vi "test_libssh2_userauth_authenticated.vi"() -> ()   [LabVIEW 2017, in "integration_tests.lvlib"]
uses:
  integration_tests.lvlib
  libssh2/libssh2_session_handshake_tcp.vi
  libssh2/libssh2_init_default.vi
  libssh2/libssh2_session_init_ex.vi
  <vilib>/Utility/tcp.llb/TCP Get Raw Net Object.vi
  libssh2/libssh2_session_handshake_socket.vi
  libssh2/libssh2_userauth_password_ex.vi
  libssh2/libssh2.lvlib
  support/support.lvlib
  <vilib>/PNR/Transparent Assertions/Transparent Assertions/Transparent Assertions.lvlib
panel:
  out "error out":errorcluster
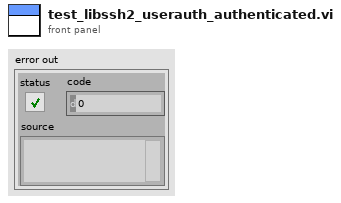
[diagram p1: front panel]
types:
  T1 = typedef "libssh2.lvlib/Session Refnum.ctl" = refnum<k1>
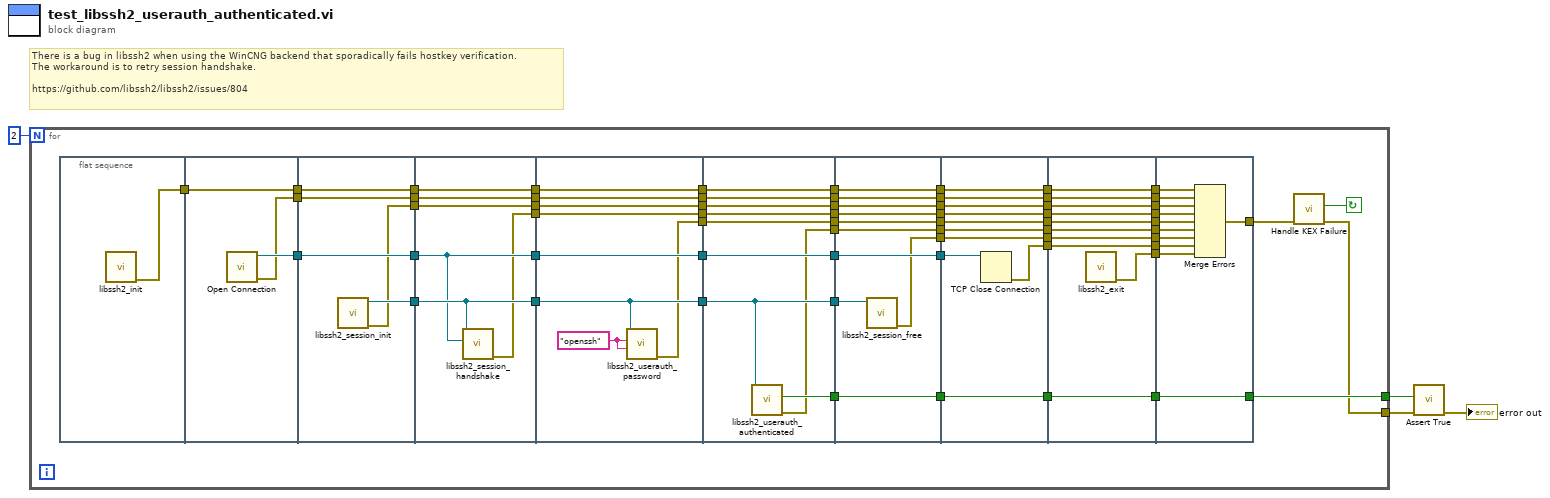
[diagram p0: block diagram]
diagram:
  # "There is a bug in libssh2 when using the WinCNG backend that sporadically fails hostkey verification.\nThe workaround is to retry session handshake.\n\nhttps://github.com/libssh2/libssh2/issues/804"
  n1 = for {
    N: 2 -> [_]
    tunnel: [w8] -> w3
    tunnel: [w5] -> w2
    stop <- w6 continue-if-true
    n2 = flat-sequence {
      tunnel: [w68] -> w67
      tunnel: [w71] -> w66
      tunnel: w67 -> [w70]
      tunnel: [w70] -> w65
      tunnel: [w69] -> w64
      tunnel: w66 -> [w76]
      tunnel: [w76] -> w63
      tunnel: w65 -> [w75]
      tunnel: [w75] -> w62
      tunnel: w64 -> [w74]
      tunnel: [w74] -> w61
      tunnel: [w73] -> w60
      tunnel: [w72] -> w59
      tunnel: w63 -> [w78]
      tunnel: [w78] -> w58
      tunnel: w62 -> [w82]
      tunnel: [w82] -> w57
      tunnel: w61 -> [w81]
      tunnel: [w81] -> w56
      tunnel: [w80] -> w55
      tunnel: w60 -> [w80]
      tunnel: w59 -> [w79]
      tunnel: [w79] -> w54
      tunnel: [w77] -> w53
      tunnel: w58 -> [w90]
      tunnel: [w90] -> w52
      tunnel: w57 -> [w89]
      tunnel: [w89] -> w51
      tunnel: w56 -> [w88]
      tunnel: [w88] -> w50
      tunnel: w55 -> [w85]
      tunnel: w54 -> [w87]
      tunnel: [w87] -> w49
      tunnel: w53 -> [w86]
      tunnel: [w86] -> w48
      tunnel: [w85] -> w47
      tunnel: [w83] -> w46
      tunnel: w52 -> [w99]
      tunnel: [w99] -> w45
      tunnel: w51 -> [w98]
      tunnel: [w98] -> w44
      tunnel: w50 -> [w97]
      tunnel: [w97] -> w43
      tunnel: w49 -> [w96]
      tunnel: [w96] -> w42
      tunnel: w48 -> [w95]
      tunnel: [w95] -> w41
      tunnel: [w92] -> w40
      tunnel: w47 -> [w93]
      tunnel: [w93] -> w39
      tunnel: w46 -> [w94]
      tunnel: [w94] -> w38
      tunnel: [w91] -> w37
      tunnel: w45 -> [w109]
      tunnel: [w109] -> w36
      tunnel: w44 -> [w108]
      tunnel: [w108] -> w35
      tunnel: w43 -> [w107]
      tunnel: [w107] -> w34
      tunnel: w42 -> [w106]
      tunnel: [w106] -> w33
      tunnel: w41 -> [w105]
      tunnel: [w105] -> w32
      tunnel: [w104] -> w31
      tunnel: [w103] -> w30
      tunnel: w40 -> [w103]
      tunnel: w39 -> [w102]
      tunnel: w38 -> [w101]
      tunnel: [w101] -> w29
      tunnel: w37 -> [w100]
      tunnel: [w100] -> w28
      tunnel: w36 -> [w119]
      tunnel: w35 -> [w118]
      tunnel: [w118] -> w27
      tunnel: w34 -> [w117]
      tunnel: [w117] -> w26
      tunnel: [w116] -> w25
      tunnel: w33 -> [w115]
      tunnel: [w115] -> w24
      tunnel: w32 -> [w114]
      tunnel: [w114] -> w23
      tunnel: [w113] -> w22
      tunnel: w31 -> [w113]
      tunnel: [w112] -> w21
      tunnel: w30 -> [w112]
      tunnel: w29 -> [w111]
      tunnel: [w111] -> w20
      tunnel: w28 -> [w110]
      tunnel: [w110] -> w19
      tunnel: w27 -> [w129]
      tunnel: [w129] -> w18
      tunnel: w26 -> [w128]
      tunnel: [w128] -> w17
      tunnel: w25 -> [w127]
      tunnel: [w127] -> w16
      tunnel: [w126] -> w15
      tunnel: w24 -> [w125]
      tunnel: [w125] -> w14
      tunnel: w23 -> [w124]
      tunnel: [w124] -> w13
      tunnel: [w123] -> w12
      tunnel: w22 -> [w123]
      tunnel: [w122] -> w11
      tunnel: w21 -> [w122]
      tunnel: w20 -> [w121]
      tunnel: [w121] -> w10
      tunnel: w19 -> [w120]
      tunnel: [w120] -> w9
      tunnel: w18 -> [w140]
      tunnel: w17 -> [w139]
      tunnel: w16 -> [w138]
      tunnel: w15 -> [w137]
      tunnel: w14 -> [w136]
      tunnel: w13 -> [w135]
      tunnel: w12 -> [w134]
      tunnel: w11 -> [w131]
      tunnel: w10 -> [w133]
      tunnel: w9 -> [w132]
      tunnel: [w131] -> w8
      tunnel: [w130] -> w7
      frame #0 {
        n3 = call-poly "libssh2_init.vi"() -> ("error out"=w68:errorcluster)  [unwired: 11 in]
      }
      frame #1 {
        n4 = call "Open Connection.vi"() -> ("error out"=w69:errorcluster, "connection ID"=w71:refnum<k5>)  [unwired: 10 in]
      }
      frame #2 {
        n5 = call "libssh2_session_init.vi"() -> ("error out"=w72:errorcluster, "session"=w73:T1)  [unwired: 10 in]
      }
      frame #3 {
        n6 = call-poly "libssh2_session_handshake.vi"("tcp connection"=w78, "session"=w80) -> ("error out"=w77:errorcluster)  [unwired: 9 in]
      }
      frame #4 {
        w84 = "openssh" ("username")
        n7 = call "libssh2_userauth_password.vi"("password"=w84, "username"=w84, "session"=w85) -> ("error out"=w83:errorcluster)  [unwired: 8 in]
      }
      frame #5 {
        n8 = call "libssh2_userauth_authenticated.vi"("session"=w93) -> ("error out"=w91:errorcluster, "authenticated"=w92:bool)  [unwired: 9 in]
      }
      frame #6 {
        n9 = call "libssh2_session_free.vi"("session"=w102) -> ("error out"=w104:errorcluster)  [unwired: 10 in]
      }
      frame #7 {
        n10 = TCP Close Connection(connection ID=w119) -> (error out=w116:errorcluster)  [unwired: 2 in, 1 out]
      }
      frame #8 {
        n11 = call "libssh2_exit.vi"() -> ("error out"=w126:errorcluster)  [unwired: 11 in]
      }
      frame #9 {
        n12 = Merge Errors(w140, w139, w136, w135, w133, w132, w134, w138, w137) -> (w130:errorcluster)
      }
    }
    n13 = call "Handle KEX Failure.vi"("error in (no error)"=w7) -> ("error out"=w5:errorcluster, "KEX Failure"=w6:bool)  [unwired: 9 in]
  }
  n14 = call <vilib>:"Assert True.vi"("error in (no error)"=w2, "Condition"=w3) -> ("error out"=→"error out":errorcluster)  [unwired: 9 in]
